vi "Register Address.vi"(8 "error in (no error)":errorcluster, 9 "Paras In":variant, 10 "ID In":variant, 11 "Simple Map Queue Group Messenger in":refnum<class "Simple Map Queue Group Messenger.lvclass">) -> (0 "error out":errorcluster, 3 "Simple Map Queue Group Messenger out":refnum<class "Simple Map Queue Group Messenger.lvclass">)   [LabVIEW 2024, in "Simple Map Queue Group Messenger.lvclass"]
uses:
  Simple Map Queue Group Messenger.lvclass
  Simple Tree Queue Messenger/Type Def/Message Queue.ctl
  Ancestor Class/Message/Message.lvclass
  Simple Map Queue Group Messenger.lvclass/Simple Map Queue Group Messenger.ctl
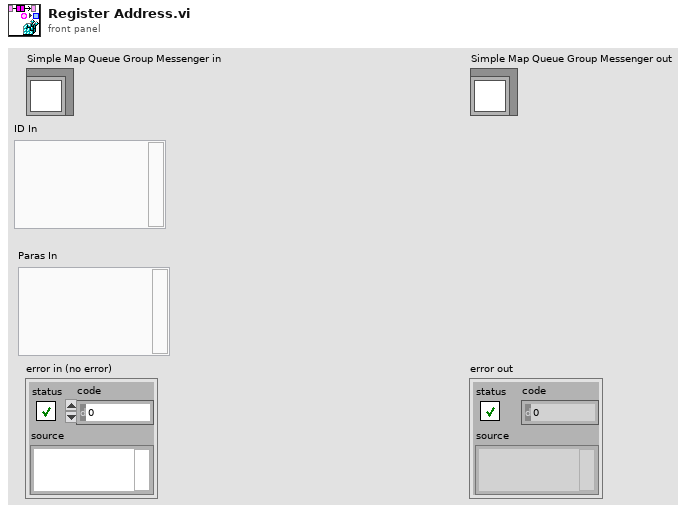
[diagram p1: front panel]
types:
  T1 = typedef "Message Queue.ctl" = refnum<queue>
  T2 = typedef "Queue Group Map.ctl" = map{i64, T1[]}
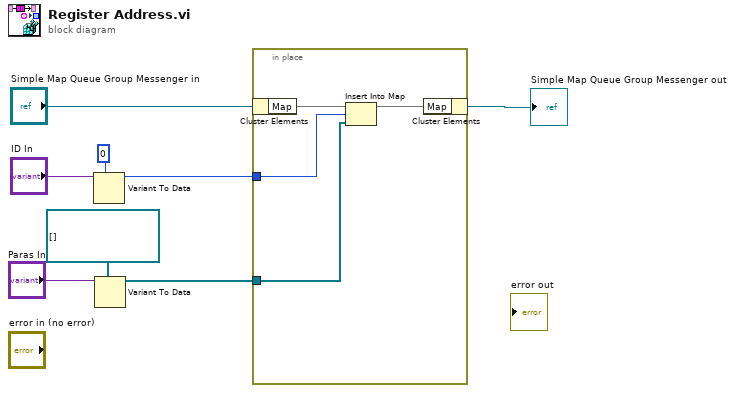
[diagram p0: block diagram]
diagram:
  n1 = Variant To Data(type=i64 0, Variant="ID In") -> (data=w4:i64)  [unwired: 1 in, 1 out]
  n2 = Variant To Data(type=T1[] [] ("value"), Variant="Paras In") -> (data=w1:T1[])  [unwired: 1 in, 1 out]
  n3 = in-place {
    in-place-border: w4 -> [w10]
    in-place-border: w1 -> [w9]
    n4 = in-place-cluster #1("Simple Map Queue Group Messenger in") -> ("Map"=w12:T2)
    n5 = Insert Into Map(map in=w12, key=w10, value=w9) -> (map out=w11:T2)  [unwired: 2 out]
    n6 = in-place-cluster #1("Map"=w11) -> (→"Simple Map Queue Group Messenger out":refnum<class "Simple Map Queue Group Messenger.lvclass">)
  }
